vi "FFT Measurement Stop.vi"(8 "error in (no error)":errorcluster, 9 "Instance (1)":i32=1, 11 "VISA resource name":refnum<visa-resource-name>) -> (0 "error out":errorcluster, 3 "VISA resource name out":refnum<visa-resource-name>)   [LabVIEW 2015, in "Rohde&Schwarz CMXP GPRF.lvlib"]
doc: "Causes a running measurement to stop after the current evaluation period is terminated and valid results are available; the R&S CMW 500 enters the \"RDY\" state.\n\nAttribute:\nRSCMXPGPRF_ATTR_FFT_MEASUREMENT_STOP\n\nRemote-control command:\nSTOP:GPRF:MEAS<i>:FFTSanalyzer"
uses:
  <instrlib>/Rohde&Schwarz CMXP GPRF/Rohde&Schwarz CMXP GPRF.lvlib
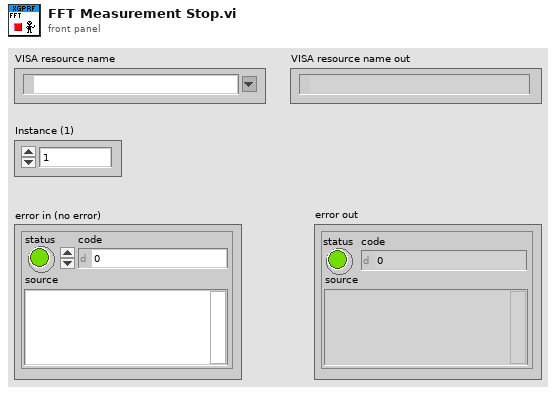
[diagram p1: front panel]
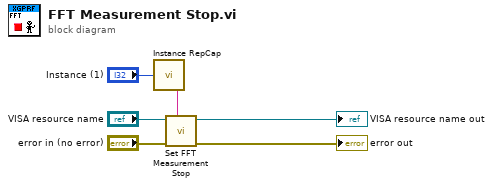
[diagram p0: block diagram]
diagram:
  n1 = call <instrlib>:"Instance RepCap.vi"("instance  in"="Instance (1)") -> ("instance out"=w6:string)
  n2 = call "Set FFT Measurement Stop"("Repeated Capabilities"=w6, "error in (no error)"="error in (no error)", "instrument handle"="VISA resource name") -> ("error out"=→"error out":errorcluster, "instrument handle out"=→"VISA resource name out":refnum<visa-resource-name>)  [unwired: 7 in]
